vi "acq_times_to_samples.vi"(10 "Acquisition Settings":T1) -> (2 "Settings to Pico":T1)   [LabVIEW 2016]
panel:
  in  "Acquisition Settings Template":T1
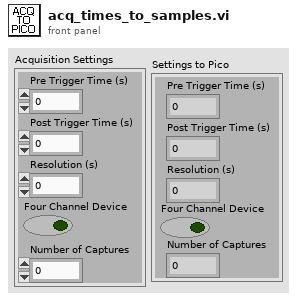
[diagram p1: front panel]
types:
  T1 = cluster{"Pre Trigger Time (s)":dbl, "Post Trigger Time (s)":dbl, "Resolution (s)":dbl, "Four Channel Device":bool, "Number of Captures":dbl}
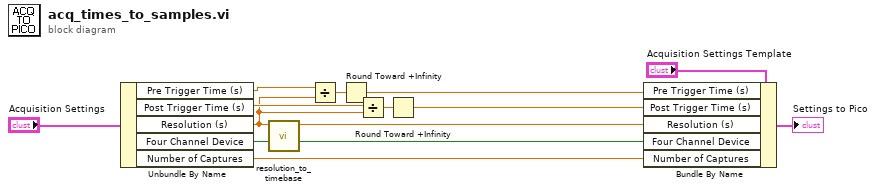
[diagram p0: block diagram]
diagram:
  n1 = Unbundle By Name("Acquisition Settings") -> ("Pre Trigger Time (s)"=w11:dbl, "Post Trigger Time (s)"=w10:dbl, "Resolution (s)"=w5:dbl, "Four Channel Device"=w12:bool, "Number of Captures"=w13:dbl)
  n2 = call "resolution_to_timebase.vi"("Resolution (s)"=w5) -> ("15 bit Timebase"=w4:dbl)  [unwired: 10 in]
  n3 = Divide(x=w11, y=w5) -> (x/y=w9:dbl)
  n4 = Round Toward +Infinity(x=w9) -> (ceil(x): smallest int >= x=w6:dbl)
  n5 = Divide(x=w10, y=w5) -> (x/y=w8:dbl)
  n6 = Round Toward +Infinity(x=w8) -> (ceil(x): smallest int >= x=w7:dbl)
  n7 = Bundle By Name(cluster="Acquisition Settings Template", "Pre Trigger Time (s)"=w6, "Post Trigger Time (s)"=w7, "Resolution (s)"=w4, "Four Channel Device"=w12, "Number of Captures"=w13) -> (→"Settings to Pico":T1)
